vi "SettingsSequence.vi"(8 "error in (no error)":errorcluster, 11 "Settings":T1) -> (0 "error out":errorcluster, 3 "Settings out":T1)   [LabVIEW 2020]
uses:
  controls/PlayerSettings.ctl
  controls/PlayerMode.ctl
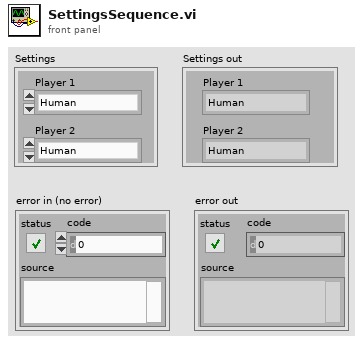
[diagram p1: front panel]
types:
  T1 = typedef "PlayerSettings.ctl" = cluster{"Player 1":T2, "Player 2":T2}
  T2 = typedef "PlayerMode.ctl" = enum16{"Human", "Bot Random", "Bot Intermidiate", "Bot Perfect Play"}
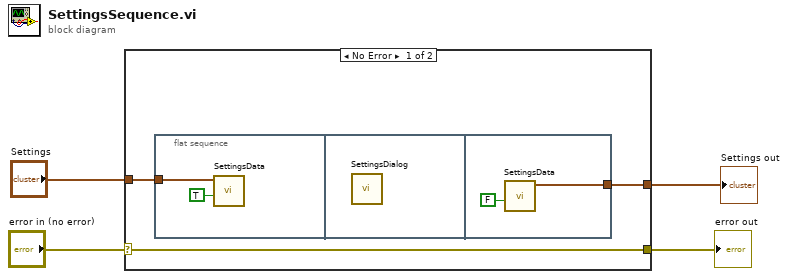
[diagram p0: block diagram]
diagram:
  n1 = case shown="No Error" "error in (no error)" {
    selector: "error in (no error)" -> [w5 w13]
    tunnel: [w7 w12] -> w4
    tunnel: "Settings" -> [w6 w12]
    tunnel: [w5 w13] -> w1
    frame No Error {
      n2 = flat-sequence {
        tunnel: w6 -> [w8]
        tunnel: [w10] -> w7
        frame #0 {
          n3 = call "SettingsData.vi"("Write (T)/Read (F)"=TRUE, "Settings in"=w8) -> ()  [unwired: 9 in, 1 out]
        }
        frame #1 {
          n4 = call "SettingsDialog.vi"() -> ()  [unwired: 12 in]
        }
        frame #2 {
          n5 = call "SettingsData.vi"("Write (T)/Read (F)"=FALSE) -> ("Settings out"=w10:T1)  [unwired: 10 in]
        }
      }
    }
    frame Error {
    }
  }
  "Settings out" <- w4
  "error out" <- w1
